vi "readMsg.vi"(0 "SPI Config In":T1) -> (2 "SPI Config Out":T1, 3 "ID":u32 format="%x", 4 "CAN Msg":u8[](array[numeric]) format="%02x", 5 "Read Data?":bool)   [LabVIEW 2019]
uses:
  SPI/SPI Config.ctl
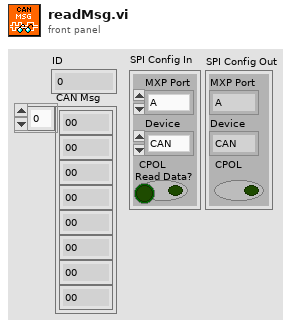
[diagram p1: front panel]
types:
  T1 = typedef "SPI Config.ctl" = cluster{"MXP Port":enum16{"A", "B"}, "Device":enum16{"CAN", "ENC", "IMU1", "IMU2"}, "CPOL":bool}
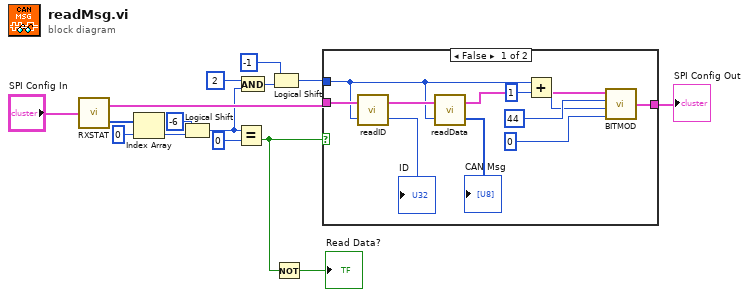
[diagram p0: block diagram]
diagram:
  n1 = call "RXSTAT.vi"("SPI Config In"="SPI Config In") -> ("SPI Config Out"=w13:T1, "Frames Read"=w12:u8[])
  n2 = Index Array(array=w12, index=0) -> (element=w10:u8)
  n3 = Logical Shift(y=i16 -6, x=w10) -> (x << y=w5:u8)
  n4 = Equal?(x=w5, y=u8 0) -> (x = y?=w6:bool)
  n5 = And(x=u8 2, y=w5) -> (x .and. y?=w3:u8)
  n6 = Logical Shift(y=i16 -1, x=w3) -> (x << y=w1:u8)
  n7 = Not(x=w6) -> (.not. x?=→"Read Data?":bool)
  n8 = case shown="False" w6 {
    tunnel: w13 -> [w22 w27]
    tunnel: [w19 w27] -> w15
    tunnel: w1 -> [w16 _]
    frame False {
      n9 = call "readID.vi"("Buffer Num"=w16, "SPI Config In"=w22) -> ("ID"=→"ID":u32, "SPI Config Out"=w21:T1)
      n10 = call "readData.vi"("Buffer Num"=w16, "SPI Config In"=w21) -> ("Data Read"=→"CAN Msg":u8[], "SPI Config Out"=w20:T1)
      n11 = Add(x=w16, y=u8 1) -> (x+y=w24:u8)
      n12 = call "BITMOD.vi"("Data"=u8 0, "Mask"=w24, "Address"=u8 44, "SPI Config In"=w20) -> ("SPI Config Out"=w19:T1)
    }
    frame True {
    }
  }
  "SPI Config Out" <- w15
